vi "VI Tree.vi"   [LabVIEW 2012, in "Phidget Voltage Ratio Input.lvlib"]
doc: "${VoltageRatioInput:VITreeHeader}"
uses:
  <instrlib>/Phidgets/Phidget Voltage Ratio Input/Phidget Voltage Ratio Input.lvlib
  <instrlib>/Phidgets/Phidget Voltage Ratio Input/Public/VoltageRatioInputStart.vi
  <instrlib>/Phidgets/Phidget Voltage Ratio Input/Public/VoltageRatioInputOpen.vi
  <instrlib>/Phidgets/Phidget Voltage Ratio Input/Public/VoltageRatioInputClose.vi
panel:
  # "(c) 2015 Phidgets Inc..  ALL RIGHTS RESERVED."
  # "SEE DIAGRAM\nFOR VI TREE."
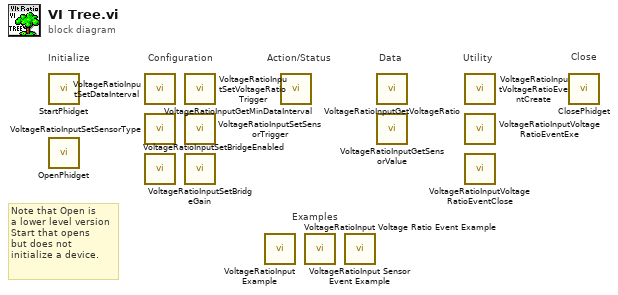
[diagram p0: block diagram]
diagram:
  # "Note that Open is\na lower level version\nStart that opens\nbut does not \ninitialize a device."
  # "Examples"
  # "Configuration"
  # "Utility"
  # "Data"
  # "Action/Status"
  # "Close"
  # "Initialize"
  n1 = call-poly <instrlib>:"StartPhidget.vi"() -> ()  [unwired: 12 in, 4 out]
  n2 = call-poly <instrlib>:"OpenPhidget.vi"() -> ()  [unwired: 8 in, 4 out]
  n3 = call <instrlib>:"VoltageRatioInputSetDataInterval.vi"() -> ()  [unwired: 9 in, 2 out]
  n4 = call <instrlib>:"VoltageRatioInputSetSensorType.vi"() -> ()  [unwired: 9 in, 2 out]
  n5 = call <instrlib>:"VoltageRatioInputSetBridgeEnabled.vi"() -> ()  [unwired: 9 in, 2 out]
  n6 = call <instrlib>:"VoltageRatioInputSetVoltageRatioTrigger.vi"() -> ()  [unwired: 9 in, 2 out]
  n7 = call <instrlib>:"VoltageRatioInputSetSensorTrigger.vi"() -> ()  [unwired: 9 in, 2 out]
  n8 = call <instrlib>:"VoltageRatioInputSetBridgeGain.vi"() -> ()  [unwired: 9 in, 2 out]
  n9 = call <instrlib>:"VoltageRatioInput Example.vi"() -> ()  [unwired: 12 in]
  n10 = call <instrlib>:"VoltageRatioInputGetMinDataInterval.vi"() -> ()  [unwired: 8 in, 3 out]
  n11 = call <instrlib>:"VoltageRatioInput Voltage Ratio Event Example.vi"() -> ()  [unwired: 12 in]
  n12 = call <instrlib>:"VoltageRatioInput Sensor Event Example.vi"() -> ()  [unwired: 12 in]
  n13 = call <instrlib>:"VoltageRatioInputGetVoltageRatio.vi"() -> ()  [unwired: 8 in, 3 out]
  n14 = call <instrlib>:"VoltageRatioInputGetSensorValue.vi"() -> ()  [unwired: 8 in, 3 out]
  n15 = call <instrlib>:"VoltageRatioInputVoltageRatioEventCreate.vi"() -> ()  [unwired: 9 in, 3 out]
  n16 = call <instrlib>:"VoltageRatioInputVoltageRatioEventExe.vi"() -> ()  [unwired: 5 in, 7 out]
  n17 = call <instrlib>:"VoltageRatioInputVoltageRatioEventClose.vi"() -> ()  [unwired: 10 in, 2 out]
  n18 = call-poly <instrlib>:"ClosePhidget.vi"() -> ()  [unwired: 11 in, 1 out]
